vi "Chemin daté AAMMJJ_SD.vi"() -> (0 "chemin du dossier":path=path "D:/111118")   [LabVIEW 2015]
panel:
  out "chemin":string="D:\\111118\\"
  out "date à l'allemande":string="111118\\"
  out "date":string="18/11/2011"
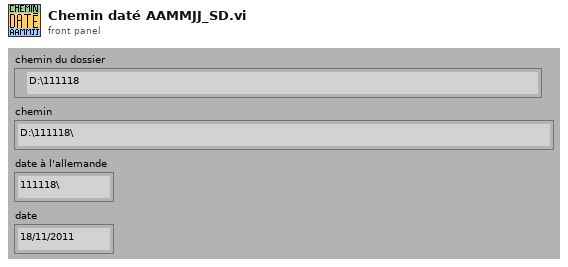
[diagram p1: front panel]
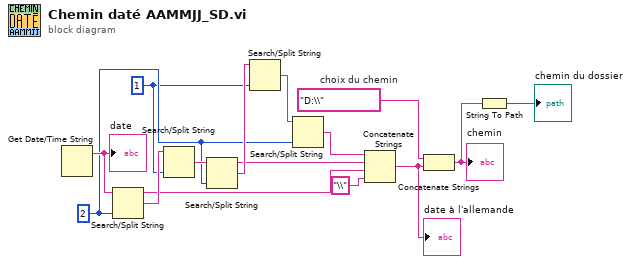
[diagram p0: block diagram]
diagram:
  w4 = "D:\\"  # choix du chemin
  w6 = 1 ("offset (0)")
  w7 = 2 ("offset (0)")
  n1 = Get Date/Time String() -> (date string=w15:string)  [unwired: 3 in, 1 out]
  "date" <- w15
  n2 = Search/Split String(string=w15, offset (0)=w7) -> (substring before match=w9:string, match + rest of string=w14:string)  [unwired: 1 in, 1 out]
  n3 = Search/Split String(string=w14, offset (0)=w6) -> (match + rest of string=w13:string)  [unwired: 1 in, 2 out]
  n4 = Search/Split String(string=w13, offset (0)=w7) -> (substring before match=w10:string, match + rest of string=w12:string)  [unwired: 1 in, 1 out]
  n5 = Search/Split String(string=w12, offset (0)=w6) -> (match + rest of string=w11:string)  [unwired: 1 in, 2 out]
  n6 = Search/Split String(string=w11, offset (0)=w7) -> (match + rest of string=w8:string)  [unwired: 1 in, 2 out]
  n7 = Concatenate Strings(w8, w10, w9, "\\" ("chaîne")) -> (w5:string)
  "date à l'allemande" <- w5
  n8 = Concatenate Strings(w4, w5) -> (w3:string)
  "chemin" <- w3
  n9 = String To Path ("Chaîne en chemin")(string=w3) -> (path=→"chemin du dossier":path)
